vi "_ClassManager_RenameMembers.vi"(8 "error in (no error)":errorcluster, 9 "ReplaceString":string, 10 "SearchString":string, 11 "LVClassLibrary Refnum":refnum<vi>) -> (0 "error out":errorcluster, 3 "Library Refnum out":refnum<vi>)   [LabVIEW 2014, in "_ClassManager.lvlib" / "_ClassManager.lvclass"]
uses:
  _ClassManager.lvclass
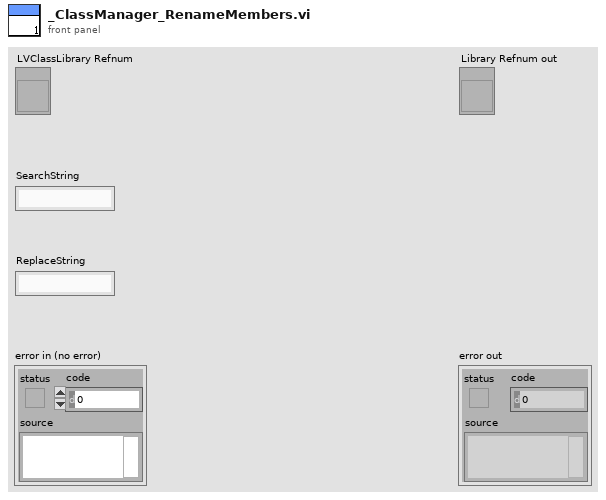
[diagram p1: front panel]
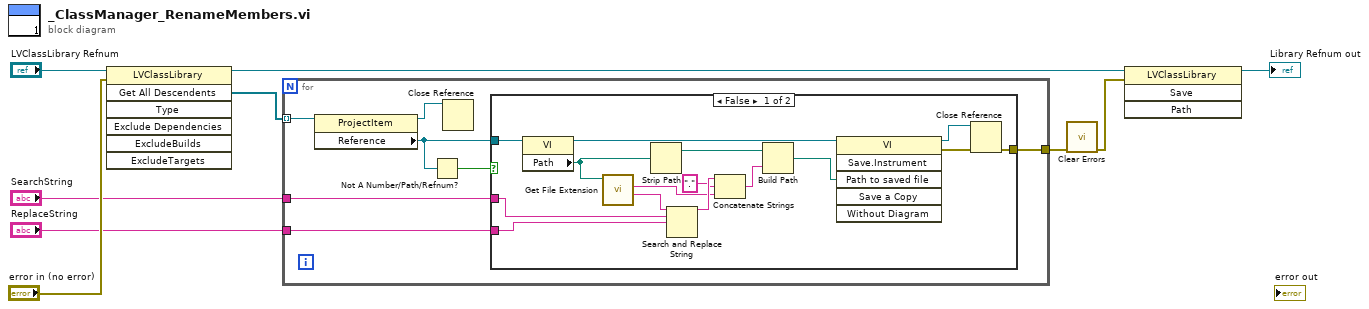
[diagram p0: block diagram]
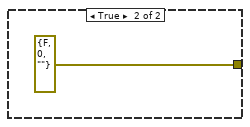
[diagram p2: hidden frame]
diagram:
  n1 = invoke class="LVClassLibrary" method="Get All Descendents"(reference="LVClassLibrary Refnum", error in="error in (no error)") -> (reference out=w8:refnum<vi>, "All Descendents"=w6:refnum<vi>[])  [unwired: 5 in, 5 out]
  n2 = for {
    tunnel: w6 -> [w16] mode=indexing
    tunnel: "SearchString" -> [w12]
    tunnel: "ReplaceString" -> [w11]
    tunnel: [w10] -> w3
    n3 = property class="ProjectItem"(reference=w16) -> (reference out=w13:refnum<vi>, "Reference"=w14:refnum<vi>)  [unwired: 1 in, 1 out]
    n4 = Not A Number/Path/Refnum?(number/path/refnum=w14) -> (NaN/Path/Refnum?=w15:bool)
    n5 = Close Reference(reference=w13) -> ()  [unwired: 1 in, 1 out]
    n6 = case shown="False" w15 {
      tunnel: w14 -> [w31 _]
      tunnel: w12 -> [w29 _]
      tunnel: w11 -> [w28 _]
      tunnel: [w18 errorcluster {"status"=FALSE, "code"=0, "source"=""} ("error out")] -> w10
      frame False {
        n7 = property class="VI"(reference=w31) -> (reference out=w27:refnum<vi>, "Path"=w26:path)  [unwired: 1 in, 1 out]
        n8 = call <vilib>:"Get File Extension.vi"("file"=w26) -> ("filename without extension"=w30:string, "lowercase file extension"=w24:string)  [unwired: 7 in, 2 out]
        n9 = Strip Path(path=w26) -> (stripped path=w23:path)  [unwired: 1 out]
        n10 = Search and Replace String(input string=w30, search string=w29, replace string=w28) -> (result string=w25:string)  [unwired: 5 in, 3 out]
        n11 = Concatenate Strings(w25, "." ("string"), w24) -> (w22:string)
        n12 = Build Path(base path=w23, name or relative path=w22) -> (appended path=w21:path)
        n13 = invoke class="VI" method="Save.Instrument"(reference=w27, "Path to saved file"=w21) -> (reference out=w19:refnum<vi>, error out=w20:errorcluster)  [unwired: 4 in, 4 out]
        n14 = Close Reference(reference=w19, error in (no error)=w20) -> (error out=w18:errorcluster)
      }
      frame True {
      }
    }
  }
  n15 = call <vilib>:"Clear Errors.vi"("error in (no error)"=w3) -> ("error out"=w1:errorcluster)  [unwired: 5 in, 1 out]
  n16 = invoke class="LVClassLibrary" method="Save"(reference=w8, error in=w1) -> (reference out=→"Library Refnum out":refnum<vi>)  [unwired: 2 in, 3 out]
